vi "readInStagesFromXML.vi"(8 "error in (no error)":errorcluster, 10 "NativeXML":refnum<class "NativeXML.lvclass">, 11 "deviceDataBase in":refnum<class "deviceDataBase.lvclass">) -> (0 "error out":errorcluster, 2 "NativeXML out":refnum<class "NativeXML.lvclass">, 3 "deviceDataBase out":refnum<class "deviceDataBase.lvclass">)   [LabVIEW 2011, in "Tools.lvlib" / "DatabaseHelpers.lvlib" / "deviceDataBase.lvclass"]
uses:
  deviceDataBase.lvclass
  NativeXML/NativeXML.lvclass
  deviceDataBase.lvclass/deviceDataBase.ctl
  <vilib>/xml/Close Reference(Node).vi
  <vilib>/xml/NI_XML.lvlib
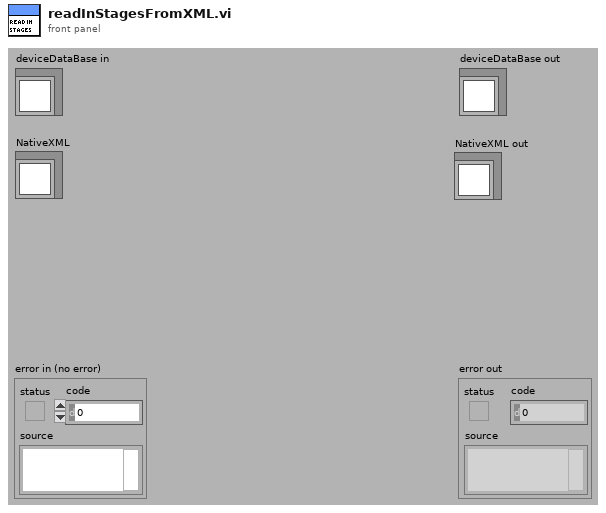
[diagram p1: front panel]
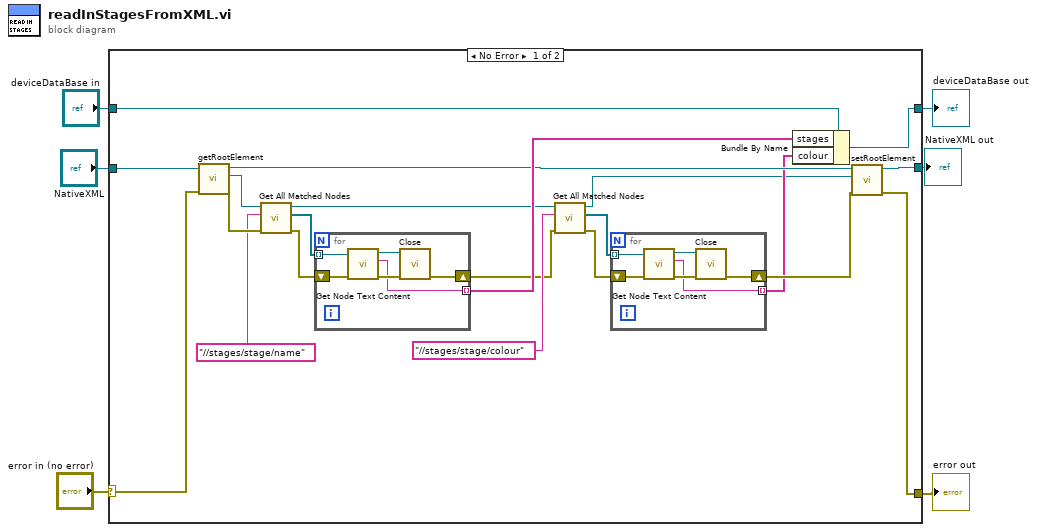
[diagram p0: block diagram]
diagram:
  n1 = case shown="No Error" "error in (no error)" {
    selector: "error in (no error)" -> [w26 w41]
    tunnel: [w16 w41] -> w5
    tunnel: [w18 w40] -> w3
    tunnel: "deviceDataBase in" -> [w19 w40]
    tunnel: "NativeXML" -> [w27 _]
    tunnel: [w15 _] -> w1
    frame No Error {
      n2 = call "getRootElement.vi"("error in (no error)"=w26, "NativeXML in"=w27) -> ("error out"=w25:errorcluster, "RootElement"=w24:refnum<k20>, "NativeXML out"=w17:refnum<class "NativeXML.lvclass">)  [unwired: 7 in]
      n3 = call <vilib>:"Get All Matched Nodes.vi"("error in (no error)"=w25, "XPath expression"="//stages/stage/name", "node in"=w24) -> ("error out"=w21:errorcluster, "node result array"=w22:refnum<k20>[], "node out"=w12:refnum<k20>)  [unwired: 6 in]
      n4 = for {
        tunnel: w22 -> [w39] mode=indexing
        tunnel: [w35] -> w20 mode=indexing
        shift-right: [w34] -> w10
        shift-left: w21 -> [w38]
        n5 = call <vilib>:"Get Node Text Content.vi"("error in (no error)"=w38, "node in"=w39) -> ("error out"=w37:errorcluster, "node text"=w35:string, "node out"=w36:refnum<k20>)  [unwired: 7 in]
        n6 = call-poly <vilib>:"Close.vi"("error in (no error)"=w37, "node"=w36) -> ("error out"=w34:errorcluster)  [unwired: 7 in]
      }
      n7 = call <vilib>:"Get All Matched Nodes.vi"("error in (no error)"=w10, "XPath expression"="//stages/stage/colour", "node in"=w12) -> ("error out"=w13:errorcluster, "node result array"=w14:refnum<k20>[], "node out"=w7:refnum<k20>)  [unwired: 6 in]
      n8 = for {
        tunnel: w14 -> [w33] mode=indexing
        tunnel: [w29] -> w8 mode=indexing
        shift-right: [w28] -> w9
        shift-left: w13 -> [w32]
        n9 = call <vilib>:"Get Node Text Content.vi"("error in (no error)"=w32, "node in"=w33) -> ("error out"=w31:errorcluster, "node text"=w29:string, "node out"=w30:refnum<k20>)  [unwired: 7 in]
        n10 = call-poly <vilib>:"Close.vi"("error in (no error)"=w31, "node"=w30) -> ("error out"=w28:errorcluster)  [unwired: 7 in]
      }
      n11 = Bundle By Name(cluster=w19, "stages"=w20, "colour"=w8) -> (w18:refnum<class "deviceDataBase.lvclass">)
      n12 = call "setRootElement.vi"("error in (no error)"=w9, "RootElement"=w7, "NativeXML in"=w17) -> ("error out"=w16:errorcluster, "NativeXML out"=w15:refnum<class "NativeXML.lvclass">)  [unwired: 7 in]
    }
    frame Error {
    }
  }
  "error out" <- w5
  "deviceDataBase out" <- w3
  "NativeXML out" <- w1
